vi "Unreserve Method.vi"(8 "error in (no error)":errorcluster, 11 "LUnit Test Case":refnum<class "LUnit Test Case V2.lvclass">) -> (0 "error out":errorcluster, 3 "LUnit Test Case 2":refnum<class "LUnit Test Case V2.lvclass">)   [LabVIEW 2020, in "LUnit Test Case V2.lvclass"]
uses:
  LUnit Test Case V2.lvclass
  LUnit Test Case V2.lvclass/LUnit Test Case V2.ctl
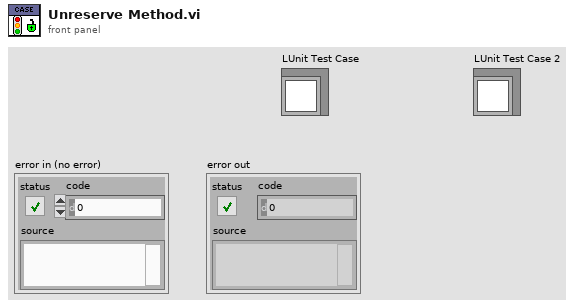
[diagram p1: front panel]
types:
  T1 = typedef "Semaphore RefNum" = refnum<k1>
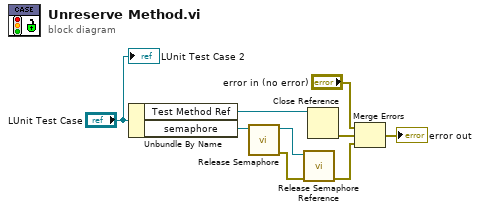
[diagram p0: block diagram]
diagram:
  n1 = Unbundle By Name("LUnit Test Case") -> ("Test Method Ref"=w8:refnum<vi>, "semaphore"=w7:T1)
  n2 = call <vilib>:"Release Semaphore.vi"("semaphore"=w7) -> ("error out"=w6:errorcluster, "semaphore out"=w5:T1)  [unwired: 5 in]
  n3 = call <vilib>:"Release Semaphore Reference.vi"("error in (no error)"=w6, "semaphore"=w5) -> ("error out"=w3:errorcluster)  [unwired: 8 in, 1 out]
  n4 = Close Reference(reference=w8) -> (error out=w9:errorcluster)  [unwired: 1 in]
  n5 = Merge Errors("error in (no error)", w9, w3) -> (→"error out":errorcluster)
  "LUnit Test Case 2" <- "LUnit Test Case"
